vi "Configure Modulation (SUM).vi"(0 "VISA resource name":refnum<visa-resource-name>, 1 "SUM Source (0: Internal)":i32(ring) items=["Internal", "External", "Channel 1", "Channel 2"], 2 "Internal Function (0: Sine)":i32(ring) items=["Sine", "Square", "RAMP", "NRAMP", "Triangle", "Noise", "PRBS", "ARB"], 5 "Channel (1: 1)":i32(ring)=1 items=["1"=1, "2"=2], 7 "Enable SUM (T: Enable)":bool=TRUE, 11 "error in (no error)":errorcluster, 12 "Modulation Depth (0.1 Percent)":dbl=0.1, 13 "SUM Internal Frequency (100 Hz)":dbl=100.0) -> (4 "VISA resource name out":refnum<visa-resource-name>, 15 "error out":errorcluster)   [LabVIEW 2019, in "Agilent 3352X Series.lvlib"]
doc: "Configures the SUM Subsystem allows you to add a modulation source signal to the primary signal on a channel. This SUM function is a simple addition of the primary signal and the SUM source signal, and it is useful for two tone generation on a single channel, or adding noise to a primary signal.\n\n<b>Note</b>:\nUse Sync Internal Phase.VI to synchronize the phase between the primary signal and the sum signal after setting the functions for primary and sum. Otherwise the phase between the two signals is arbitrary."
uses:
  <instrlib>/Agilent 3352X Series/Agilent 3352X Series.lvlib
panel:
  # "Internal SUM Modulation Settings"
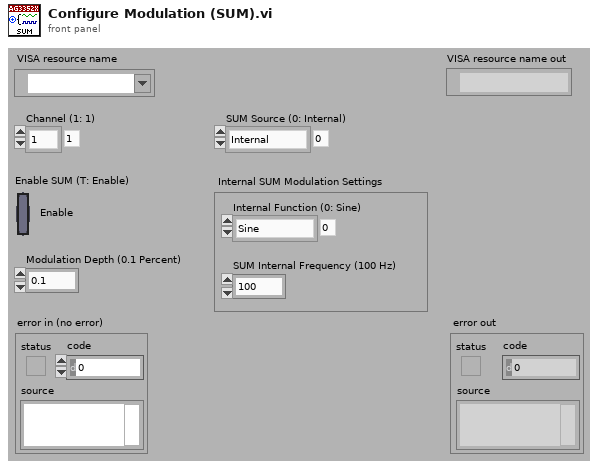
[diagram p1: front panel]
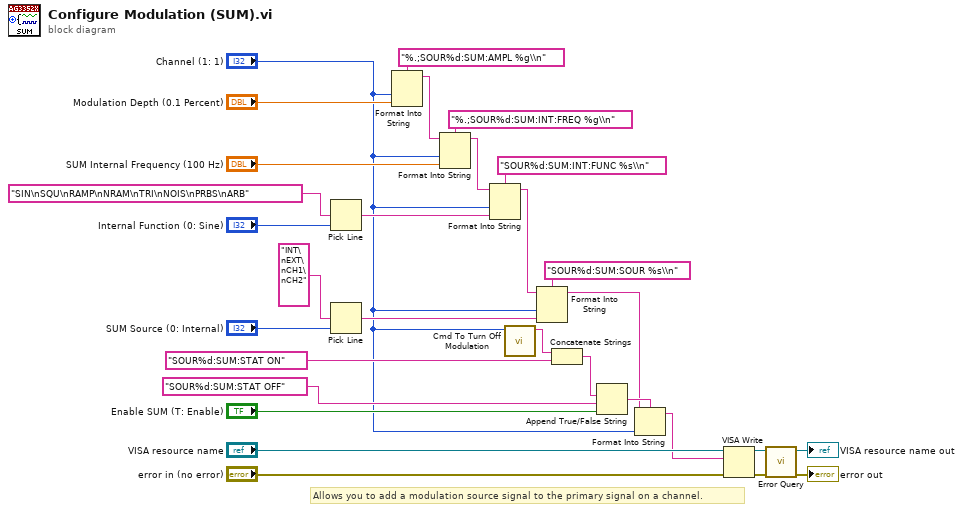
[diagram p0: block diagram]
diagram:
  # "Allows you to add a modulation source signal to the primary signal on a channel."
  n1 = Pick Line(multi-line string="SIN\nSQU\nRAMP\nNRAM\nTRI\nNOIS\nPRBS\nARB", line index="Internal Function (0: Sine)") -> (output string=w12:string)  [unwired: 1 out]
  n2 = Pick Line(multi-line string="INT\nEXT\nCH1\nCH2", line index="SUM Source (0: Internal)") -> (output string=w14:string)  [unwired: 1 out]
  n3 = Format Into String(format string="%.;SOUR%d:SUM:AMPL %g\\n", "Channel (1: 1)", "Modulation Depth (0.1 Percent)") -> (resulting string=w29:string)  [unwired: 2 in, 1 out]
  n4 = Format Into String(format string="%.;SOUR%d:SUM:INT:FREQ %g\\n", initial string=w29, "Channel (1: 1)", "SUM Internal Frequency (100 Hz)") -> (resulting string=w26:string)  [unwired: 1 in, 1 out]
  n5 = Format Into String(format string="SOUR%d:SUM:INT:FUNC %s\\n", initial string=w26, "Channel (1: 1)", w12) -> (resulting string=w24:string)  [unwired: 1 in, 1 out]
  n6 = call <instrlib>:"Cmd To Turn Off Modulation.vi"("Channel (1: 1)"="Channel (1: 1)") -> ("Cmd String"=w6:string)  [unwired: 10 out]
  n7 = Format Into String(format string="SOUR%d:SUM:SOUR %s\\n", initial string=w24, "Channel (1: 1)", w14) -> (resulting string=w3:string)  [unwired: 1 in, 1 out]
  n8 = Concatenate Strings(w6, "SOUR%d:SUM:STAT ON") -> (w9:string)
  n9 = Append True/False String(1:"Enable SUM (T: Enable)", 2:"SOUR%d:SUM:STAT OFF", 3:w9) -> (0:w8:string)  [unwired: 1 out]
  n10 = Format Into String(format string=w8, initial string=w3, "Channel (1: 1)") -> (resulting string=w2:string)  [unwired: 1 in, 1 out]
  n11 = VISA Write(VISA resource name="VISA resource name", write buffer=w2, error in (no error)="error in (no error)") -> (VISA resource name out=w20:refnum<visa-resource-name>, error out=w19:errorcluster)  [unwired: 1 out]
  n12 = call <instrlib>:"Error Query.vi"("error in (no error)"=w19, "VISA resource name"=w20) -> ("error out"=→"error out":errorcluster, "VISA resource name out"=→"VISA resource name out":refnum<visa-resource-name>)  [unwired: 8 out]
